vi "New Subscription Request.vi"(8 "Subscription Policy":T1, 9 "Subscriber ID":string, 10 "Type":variant, 11 "Datum Name":string) -> (3 "SubscriptionRequest":refnum<class "SubscriptionRequest.lvclass">)   [LabVIEW 2015, in "IMediator.lvlib" / "SubscriptionRequest.lvclass"]
doc: "<License>\nCopyright © 2017 Composed Systems, LLC | All rights reserved\nwww.composed.io\n\nAuthor: Ethan Stern <ethan.stern@composed.io>\n\nThis software is provided \"AS IS\" WITHOUT WARRANTIES, either express or implied, AND IS FOR EDUCATIONAL PURPOSES ONLY.\n</License>"
uses:
  SubscriptionRequest.lvclass
  ISubscriptionPolicy/ISubscriptionPolicy Reference.ctl
  ISubscriptionPolicy/ISubscriptionPolicy.lvclass
  SubscriptionRequest.lvclass/SubscriptionRequest.ctl
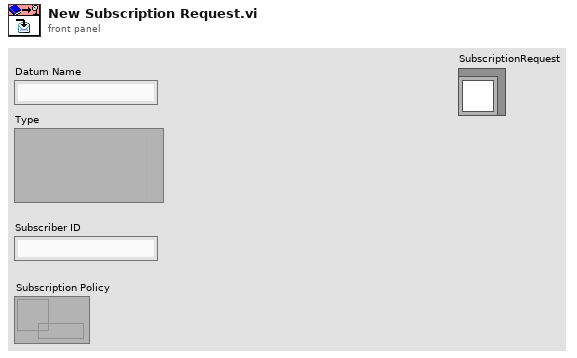
[diagram p1: front panel]
types:
  T1 = typedef "IMediator.lvlib/ISubscriptionPolicy.lvclass/ISubscriptionPolicy Reference.ctl" = refnum<data-value>
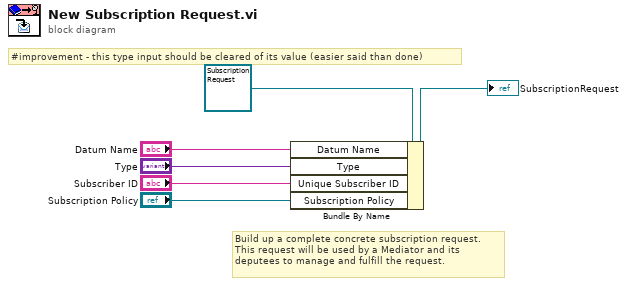
[diagram p0: block diagram]
diagram:
  # "Build up a complete concrete subscription request.\nThis request will be used by a Mediator and its\ndeputees to manage and fulfill the request."
  # "#improvement - this type input should be cleared of its value (easier said than done)"
  n1 = Bundle By Name(cluster=refnum<class "SubscriptionRequest.lvclass"> refnum ("SubscriptionRequest in"), "Datum Name"="Datum Name", "Type"="Type", "Unique Subscriber ID"="Subscriber ID", "Subscription Policy"="Subscription Policy") -> (→"SubscriptionRequest":refnum<class "SubscriptionRequest.lvclass">)
